vi "Launch uService.vi"(6 "uService ID (optional)":string, 8 "error in (no error)":errorcluster, 9 "GUI?":bool, 10 "Class Name":string, 11 "Father of all uServices in":refnum<class "Father of all uServices.lvclass">) -> (0 "error out":errorcluster, 3 "Father of all uServices out":refnum<class "Father of all uServices.lvclass">)   [LabVIEW 2026, in "TALOS.lvlib" / "Father of all uServices.lvlib" / "Father of all uServices.lvclass"]
doc: "Use this VI to programmatically launch a µService. Be sure to provide a way to shutdown the µService launched (internal, or via a message)! If you don't need to display any GUI for this µService, mark the connector GUI? as False. By default, the uService Class Name is used as ID: if something is specified in \"uService ID (optional)\", then that sting is used as ID (useful, for example, for launching multiple istances of the same uService)."
uses:
  Father of all uServices.lvclass
  C:/LabVIEW Code/TALOS/builds/Actor Framework PPL/Actor Framework.lvlibp/1abvi3w/vi.lib/ActorFramework/Actor/Actor.lvclass
  Guardian/Guardian Messages/Launch uService Msg/Launch uService Msg.lvclass/Launch uService Msg.ctl
  Ancestor/Ancestor/Ancestor.lvclass/Ancestor.ctl
  Support VIs/Generate Error.vi
  FGV/Error Memory/Get Error Description.vi
  Support VIs/Get PC name.vi
  Ancestor/Ancestor/Read ID.vi
  Support VIs/Get Class Name.vi
  <vilib>/Utility/error.llb/Clear Errors.vi
  FGV/Error Memory/Error Memory Core.vi
  <vilib>/AdvancedString/Delimited String to 1D String Array.vi
  <vilib>/AdvancedString/Delimited String to 1D String Array (string).vi
  Support VIs/Circus Root Path.vi
  FGV/Error Memory/Error Crt Lvl checker.vi
  FGV/Error Memory/Error Memory Core.vi/40c8088d-b597-4017-91af-faa98e00292e.vi
  FGV/Error Memory/Error Memory Core.vi/d4a3ab98-063c-4e44-b43d-fbdcfe6c2be2.vi
  builds/Actor Framework PPL/Actor Framework.lvlibp/1abvi3w/vi.lib/ActorFramework/Message Enqueuer/Enqueue.vi
  Support VIs/Global Memory.vi
  <vilib>/Utility/LVClass/Get LV Class Name.vi
  Support VIs/Is in Packed Library.vi
  Support VIs/TALOS Root path.vi
  Support VIs/Read CSV worksheet.vi
  Support VIs/Global Constants.vi
  <vilib>/Utility/error.llb/General Error Handler.vi
  Support VIs/Error Log.vi
  Guardian/Guardian Messages/Launch uService Msg/Launch uService Msg.lvclass
  Ancestor/Ancestor/Ancestor.lvclass
  <vilib>/Comparison/Equal/Equal Functor/Equal Functor.lvclass
  builds/Actor Framework PPL/Actor Framework.lvlibp/1abvi3w/vi.lib/ActorFramework/Actor/Actor.lvclass
  TALOS.lvlib
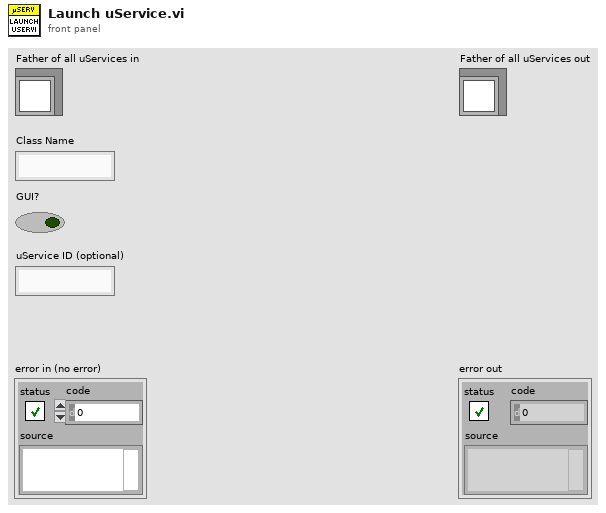
[diagram p1: front panel]
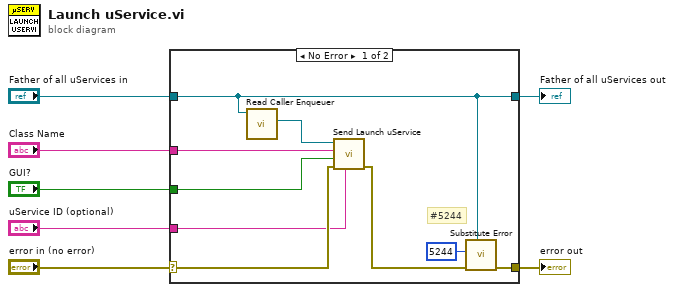
[diagram p0: block diagram]
diagram:
  n1 = case shown="No Error" "error in (no error)" {
    selector: "error in (no error)" -> [w13 w18]
    tunnel: [w11 w18] -> w6
    tunnel: [w9 w17] -> w4
    tunnel: "Father of all uServices in" -> [w9 w17]
    tunnel: "Class Name" -> [w15 _]
    tunnel: "GUI?" -> [w14 _]
    tunnel: "uService ID (optional)" -> [w12 _]
    frame No Error {
      # "#5244"
      n2 = call "Read Caller Enqueuer.vi"("Actor"=w9) -> ("Caller Enqueuer"=w16:refnum<class "Message Enqueuer.lvclass">)  [unwired: 10 in]
      n3 = call "Send Launch uService.vi"("uService ID"=w12, "error in (no error)"=w13, "GUI?"=w14, "uService Class Name"=w15, "Message Enqueuer"=w16) -> ("error out"=w10:errorcluster)  [unwired: 5 in, 1 out]
      n4 = call "Substitute Error.vi"("LabVIEW Object"=w9, "error in (no error)"=w10, "Error Code"=5244) -> ("error out"=w11:errorcluster)  [unwired: 8 in]
    }
    frame Error {
    }
  }
  "error out" <- w6
  "Father of all uServices out" <- w4
